vi "Shift And Rotation.vi"() -> ()   [LabVIEW 2014]
doc: "Use this template to build a VI to use as a subVI."
uses:
  <vilib>/vision/NI_Vision_Development_Module.lvlib
panel:
  out "Img Display":T1(plugin-control)
  # ":: MVi Framework V1.0 ::\nAuthor:Gaoke Yang\nEmail: gaoke.yang@yahoo.com\nWeb: www.mvicontrol.com\nCopyright (C) 2015, MVI Technologies All Rights Reserved"
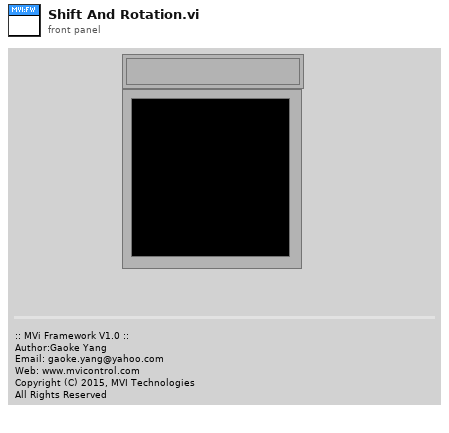
[diagram p1: front panel]
types:
  T1 = typedef "IMAQ Image.ctl" = refnum<image>
  T2 = typedef "Image Type" = u32
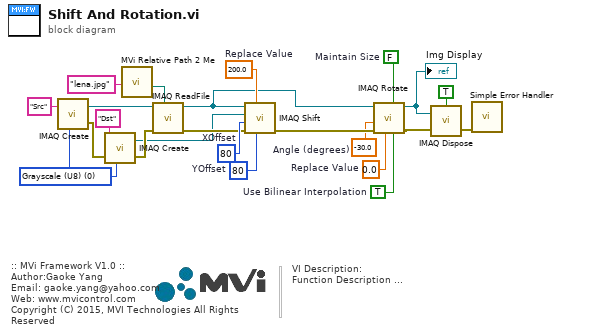
[diagram p0: block diagram]
diagram:
  w3 = FALSE  # Maintain Size
  w4 = TRUE  # Use Bilinear Interpolation
  w5 = sgl 0.0  # Replace Value
  w6 = sgl 200.0  # Replace Value
  w10 = sgl -30.0  # Angle (degrees)
  w11 = 80  # YOffset
  w12 = 80  # XOffset
  w17 = T2 0 items=["Grayscale (U8)", "Grayscale (I16)", "Grayscale (SGL)", "Complex (CSG)", "RGB (U32)", "HSL (U32)", "RGB (U64)", "Grayscale (U16)"] ("Image Type")
  # "VI Description:\nFunction Description ..."
  # ":: MVi Framework V1.0 ::\nAuthor:Gaoke Yang\nEmail: gaoke.yang@yahoo.com\nWeb: www.mvicontrol.com\nCopyright (C) 2015, MVI Technologies All Rights Reserved"
  n1 = call "IMAQ Create"("Image Name"="Src" ("name or relative path"), "Image Type"=w17) -> ("New Image"=w14:T1, "error out"=w16:errorcluster)  [unwired: 2 in, 1 out]
  n2 = call "IMAQ Create"("Image Name"="Dst" ("name or relative path"), "Image Type"=w17, "error in (no error)"=w16) -> ("New Image"=w7:T1, "error out"=w15:errorcluster)  [unwired: 1 in, 1 out]
  n3 = call "MVi Relative Path 2 Me.vi"("Relative Path"="lena.jpg" ("name or relative path")) -> ("Appended Dir"=w19:path)  [unwired: 5 in, 1 out]
  n4 = call "IMAQ ReadFile"("File Path"=w19, "error in (no error)"=w15, "Image"=w14) -> ("error out"=w8:errorcluster, "Image Out"=w1:T1)  [unwired: 4 in, 3 out]
  n5 = call "IMAQ Shift"("YOffset"=w11, "Replace Value"=w6, "error in (no error)"=w8, "XOffset"=w12, "Image Dst"=w7, "Image Src"=w1) -> ("error out"=w13:errorcluster)  [unwired: 4 in, 1 out]
  n6 = call "IMAQ Rotate"("Use Bilinear Interpolation"=w4, "Maintain Size"=w3, "Replace Value"=w5, "error in (no error)"=w13, "Angle (degrees)"=w10, "Image Src"=w1) -> ("error out"=w9:errorcluster, "Image Dst Out"=w2:T1)  [unwired: 4 in]
  "Img Display" <- w2
  n7 = call "IMAQ Dispose"("All Images? (No)"=TRUE, "Image"=w2, "error in (no error)"=w9) -> ("error out"=w20:errorcluster)  [unwired: 3 out]
  n8 = call <vilib>:"Simple Error Handler.vi"("error in (no error)"=w20) -> ()  [unwired: 1 in, 8 out]
